vi "TS_SeqBuilder.vi"(0 "Engine Ref":refnum<k7>, 5 "Steps array":T1[](array[typedef]), 7 "Test Sequence File (Save As)":string, 11 "error in":errorcluster) -> (15 "error out":errorcluster)   [LabVIEW 2011]
doc: "This VI reads a \"logical\" step array and builds a TestStand sequence from it."
uses:
  SeqBuilder/Ctls/SeqStepTypeDef.ctl
  TestComponents.ctl
  FilePaths.ctl
  Progress.vi
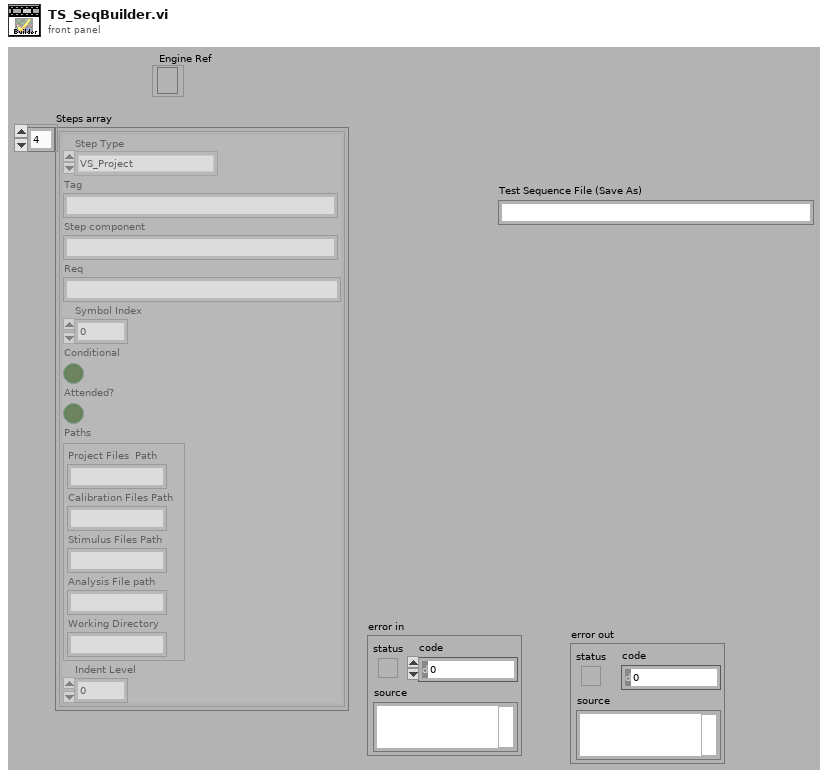
[diagram p1: front panel]
types:
  T1 = typedef "SeqStepTypeDef.ctl" = cluster{"Step Type":T2, "Tag":string, "Step component":string, "Req":string, "Symbol Index":i32, "Conditional":bool, "Attended?":bool, "Paths":T3, "Indent Level":i32}
  T2 = typedef "TestComponents.ctl" = enum16{"Script", "Test Procedure", "VS_Project", "Calibration File", "Stimulus Profile", "Analysis Script"}
  T3 = typedef "FilePaths.ctl" = cluster{"Project Files  Path":string, "Calibration Files Path":string, "Stimulus Files Path":string, "Analysis File path":string, "Working Directory":string}
  T4 = typedef "dotNetAssemblyInfo.ctl" = cluster{"VeriStand.exe Path":string, "Assembly":string, "Constructor Token":i32, "Module Token":T5}
  T5 = typedef "VSModuleTokens.ctl" = cluster{"GetIWorkspaceToken":i32, "GetIStimulusToken":i32, "GetIModelManagerToken":i32, "GetIProjectToken":i32, "RunProjectToken":i32, "CloseProjectToken":i32, "RunWorkspaceToken":i32, "StopWorkspaceToken":i32, "SetSingleChannelToken":i32, "SetMultipleParametersToken":i32, "RunStimulusToken":i32, "GetStimulusStateToken":i32, "Open WorkspaceToken":i32, "DeployToken":i32, "UndeployToken":i32, "QuitToken":i32}
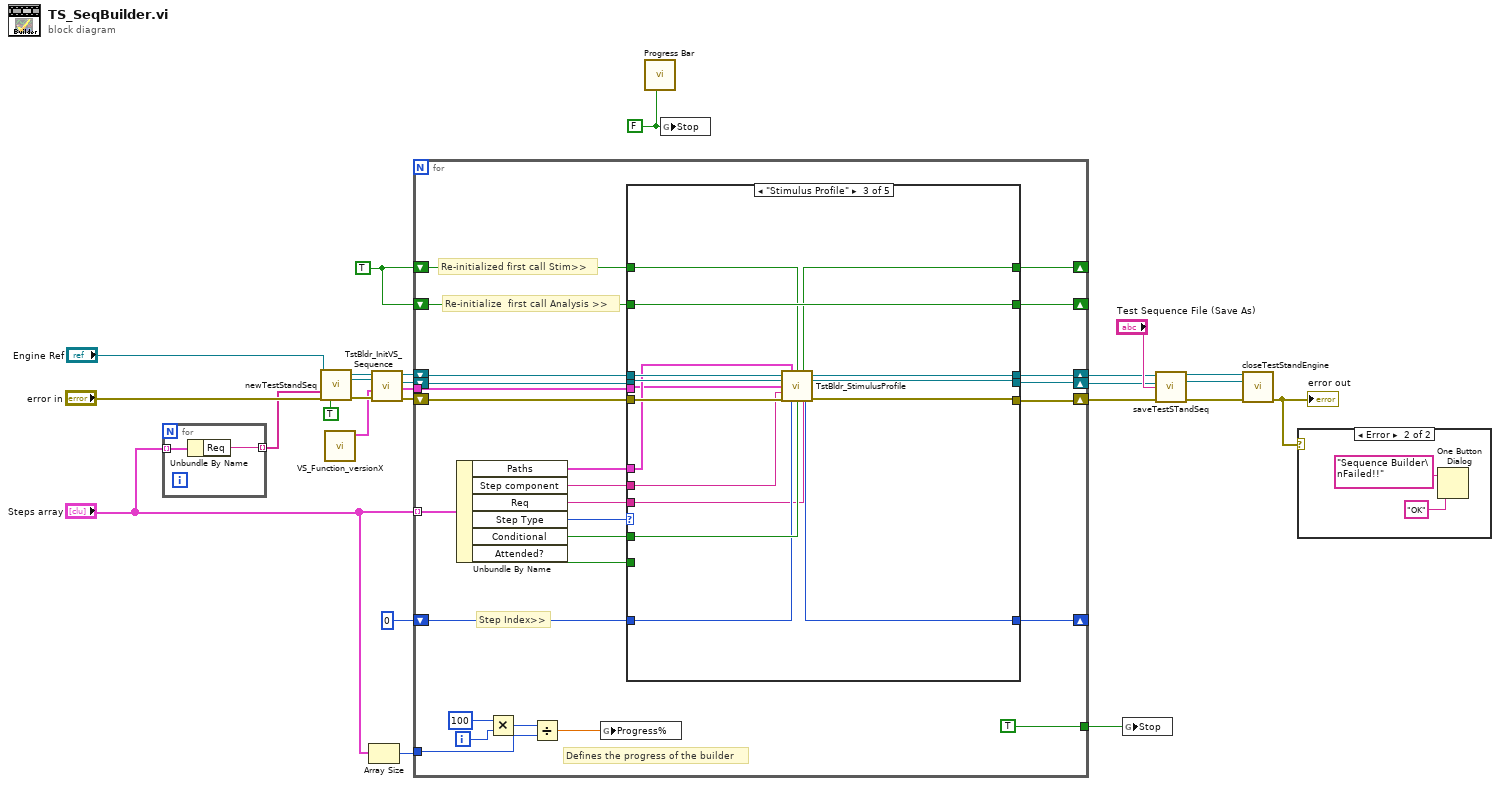
[diagram p0: block diagram]
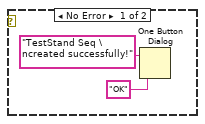
[diagram p2: hidden frame]
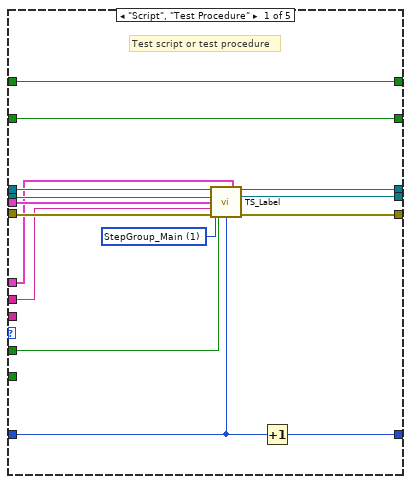
[diagram p3: hidden frame]
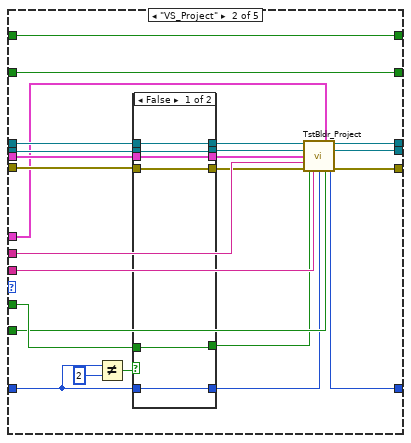
[diagram p4: hidden frame]
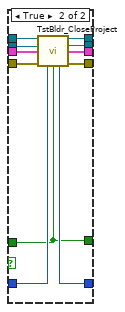
[diagram p5: hidden frame]
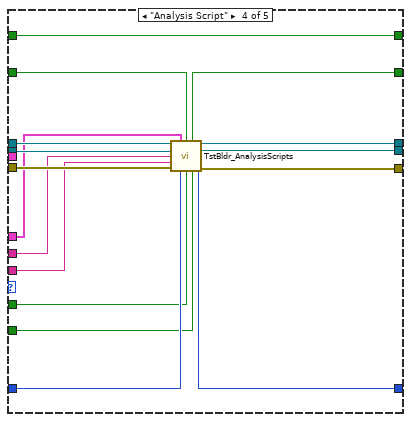
[diagram p6: hidden frame]
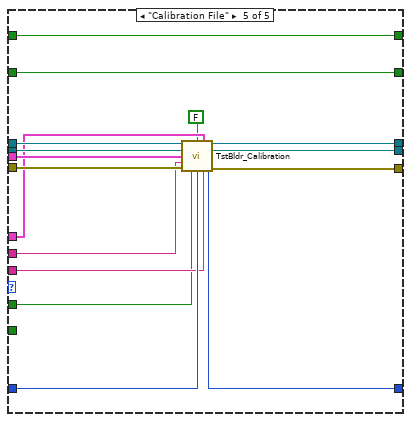
[diagram p7: hidden frame]
diagram:
  w4 = TRUE
  w3 = FALSE ("Stop")
  n1 = for {
    tunnel: "Steps array" -> [w28] mode=indexing
    tunnel: [w27] -> w14 mode=indexing
    n2 = Unbundle By Name(w28) -> ("Req"=w27:string)
  }
  n3 = call "newTestStandSeq.vi"("Engine Ref"="Engine Ref", "Requirements"=w14, "error in (no error)"="error in", "Add Req"=TRUE) -> ("Engine Reference(out)"=w20:refnum<k7>, "Sequence File Ref(out)"=w19:refnum<k7>, "error out"=w21:errorcluster)  [unwired: 9 in]
  n4 = call "VS_Function_versionX.vi"() -> ("VeriStand version info"=w2:T4)  [unwired: 11 in]
  n5 = Array Size(array="Steps array") -> (size(s)=w9:i32)
  n6 = call "TstBldr_InitVS_Sequence.vi"("error in"=w21, "VeriStand version info"=w2, "Sequence File Ref"=w19, "Engine Reference"=w20) -> ("error out"=w16:errorcluster, "VeriStand version info (out)"=w1:T4, "Sequence File Ref(out)"=w17:refnum<k7>, "Engine reference(out)"=w18:refnum<k7>)  [unwired: 4 in]
  n7 = for {
    tunnel: "Steps array" -> [w54] mode=indexing
    shift-right: [w51] -> w12
    shift-left: w18 -> [w53]
    shift-right: [w50] -> w11
    shift-left: w17 -> [w52]
    shift-right: [w48] -> w10
    shift-left: w16 -> [w49]
    shift-right: [w44] -> _
    shift-left: 0 ("Sequence index") -> [w45]
    tunnel: w9 -> [w39]
    tunnel: [TRUE ("Stop")] -> w8
    shift-right: [w34] -> _
    shift-left: w4 -> [w35]
    shift-right: [w32] -> _
    shift-left: w4 -> [w33]
    tunnel: w1 -> [w30]
    i -> [w42]
    # "Re-initialize  first call Analysis >>"
    # "Re-initialized first call Stim>>"
    # "Step Index>>"
    # "Defines the progress of the builder"
    n8 = Unbundle By Name(w54) -> ("Paths"=w29:T3, "Step component"=w46:string, "Req"=w47:string, "Step Type"=w43:T2, "Conditional"=w36:bool, "Attended?"=w31:bool)
    n9 = Multiply(x=100, y=w42) -> (x*y=w40:i32)
    n10 = Divide(x=w40, y=w39) -> (x/y=w38:dbl)
    n11 = global write "Progress.vi" "Progress%"(w38) -> ()
    n12 = case shown="\"Stimulus Profile\"" w43 {
      tunnel: w53 -> [w66 w93 w120 w140 w158]
      tunnel: w52 -> [w65 w92 w119 w139 w153]
      tunnel: [w57 w91 w117 w138 w155] -> w51
      tunnel: [w58 w90 w118 w137 w154] -> w50
      tunnel: w49 -> [w63 w89 w122 w142 w157]
      tunnel: [w59 w88 w121 w141 w156] -> w48
      tunnel: w47 -> [_ w87 w113 w133 w149]
      tunnel: w46 -> [w62 w84 w112 w134 w147]
      tunnel: w45 -> [w61 w86 w116 w136 w150]
      tunnel: [w69 w85 w115 w135 w144] -> w44
      tunnel: w36 -> [w56 w83 w123 w132 w146]
      tunnel: w35 -> [w68 w82 w125 w129 w152]
      tunnel: [w68 w82 w124 w129 w152] -> w34
      tunnel: w33 -> [w67 w81 w126 w128 w151]
      tunnel: [w67 w81 w126 w127 w151] -> w32
      tunnel: w31 -> [_ w80 _ w131 _]
      tunnel: w30 -> [w64 w79 w111 _ w148]
      tunnel: w29 -> [w55 w70 w114 w130 w145]
      frame "Script", "Test Procedure" {
        w60 = 1 items=["StepGroup_Setup", "StepGroup_Main", "StepGroup_Cleanup"] ("Step Group")
        # "Test script or test procedure"
        n13 = call "TS_Label.vi"("Engine Reference(in)"=w66, "Condition Run?"=w56, "Paths"=w55, "Sequence File Ref(in)"=w65, "VeriStand version info"=w64, "Script Name"=w62, "error in"=w63, "Step Group"=w60, "index"=w61) -> ("Engine reference(out)"=w57:refnum<k7>, "Sequence File Ref(out)"=w58:refnum<k7>, "error out"=w59:errorcluster)  [unwired: 3 in, 1 out]
        n14 = Increment(x=w61) -> (x+1=w69:i32)
      }
      frame "VS_Project" {
        n15 = Not Equal?(x=w86, y=2) -> (x != y?=w77:bool)
        n16 = case shown="False" w77 {
          tunnel: w86 -> [w99 w104]
          tunnel: [w99 w103] -> w73
          tunnel: w93 -> [w98 w110]
          tunnel: [w98 w109] -> w76
          tunnel: w92 -> [w97 w108]
          tunnel: [w97 w107] -> w75
          tunnel: w89 -> [w96 w106]
          tunnel: [w96 w105] -> w74
          tunnel: w83 -> [w95 w102]
          tunnel: [w95 w102] -> w72
          tunnel: w79 -> [w94 w101]
          tunnel: [w94 w100] -> w71
          frame False {
          }
          frame True {
            n17 = call "TstBldr_CloseProject.vi"("Engine reference"=w110, "Sequence File Ref"=w108, "VeriStand version info"=w101, "error in"=w106, "Sequence index"=w104, "Condition run?"=w102) -> ("Engine reference (out)"=w109:refnum<k7>, "Sequence File Ref(out)"=w107:refnum<k7>, "VeriStand version info (out)"=w100:T4, "Sequence index out"=w103:i32, "error out"=w105:errorcluster)  [unwired: 5 in]
          }
        }
        n18 = call "TstBldr_Project.vi"("Engine reference"=w76, "Condition run?"=w72, "Paths"=w70, "Sequence File Ref"=w75, "VeriStand version info"=w71, "Project Name"=w84, "error in"=w74, "Requirement"=w87, "Sequence index"=w73, "Attended?"=w80) -> ("Engine reference (out)"=w91:refnum<k7>, "Sequence File Ref(out)"=w90:refnum<k7>, "Sequence index out"=w85:i32, "error out"=w88:errorcluster)  [unwired: 2 in]
      }
      frame "Stimulus Profile" {
        n19 = call "TstBldr_StimulusProfile.vi"("Engine reference"=w120, "Paths"=w114, "First call?"=w125, "Sequence File Ref"=w119, "VeriStand version info"=w111, "Step Name"=w112, "error in"=w122, "Sequence index"=w116, "Condition Run?"=w123, "Requirement"=w113) -> ("First call? out"=w124:bool, "Engine reference (out)"=w117:refnum<k7>, "Sequence File Ref(out)"=w118:refnum<k7>, "Sequence index (out)"=w115:i32, "error out"=w121:errorcluster)  [unwired: 1 in]
      }
      frame "Analysis Script" {
        n20 = call "TstBldr_AnalysisScripts.vi"("Engine reference"=w140, "paths"=w130, "First call?"=w128, "Sequence File Ref"=w139, "Step Name"=w134, "Requirement"=w133, "error in"=w142, "Sequence index"=w136, "Conition Run?"=w132, "Attended?"=w131) -> ("First call? out"=w127:bool, "Engine reference (out)"=w138:refnum<k7>, "Sequence File Ref(out)"=w137:refnum<k7>, "Sequence index (out)"=w135:i32, "error out"=w141:errorcluster)  [unwired: 1 in]
      }
      frame "Calibration File" {
        n21 = call "TstBldr_Calibration.vi"("Engine reference"=w158, "m file?"=FALSE, "Paths"=w145, "Sequence File Ref"=w153, "VeriStand version info"=w148, "Step Name"=w147, "error in"=w157, "Conditional Run?"=w146, "Sequence index"=w150, "Requirement"=w149) -> ("Engine reference (out)"=w155:refnum<k7>, "Sequence File Ref(out)"=w154:refnum<k7>, "Sequence index (out)"=w144:i32, "error out"=w156:errorcluster)  [unwired: 2 in]
      }
    }
  }
  n22 = call "Progress Bar.vi"("Multiple files?"=w3) -> ()  [unwired: 11 in]
  n23 = global write "Progress.vi" "Stop"(w3) -> ()
  n24 = global write "Progress.vi" "Stop"(w8) -> ()
  n25 = call "saveTestSTandSeq.vi"("Engine reference"=w12, "Sequence File Ref"=w11, "pathString"="Test Sequence File (Save As)", "error in"=w10) -> ("Engine reference(out)"=w6:refnum<k7>, "Sequence File Ref(out)"=w7:refnum<k7>, "error out"=w5:errorcluster)  [unwired: 9 in]
  n26 = call "closeTestStandEngine.vi"("error in (no error)"=w5, "Sequence File Ref"=w7, "Engine Reference"=w6) -> ("error out"=w26:errorcluster)  [unwired: 8 in]
  "error out" <- w26
  n27 = case shown="Error" w26 {
    frame No Error {
      n28 = One Button Dialog(message="TestStand Seq \ncreated successfully!", button name ("OK")="OK") -> ()  [unwired: 1 out]
    }
    frame Error {
      n29 = One Button Dialog(message="Sequence Builder\nFailed!!", button name ("OK")="OK") -> ()  [unwired: 1 out]
    }
  }
